vi "Finished Parsing an Array.vi"(11 "JSON Parser in":refnum<class "JSON Parser.lvclass">) -> (3 "JSON Parser out":refnum<class "JSON Parser.lvclass">)   [LabVIEW 2020, in "JKI JSON Serialization.lvlib" / "JSON Parser.lvclass"]
uses:
  JSON Parser.lvclass
  JSON Parser.lvclass/JSON Parser.ctl
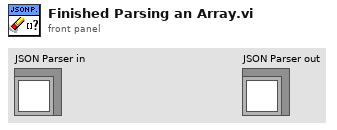
[diagram p1: front panel]
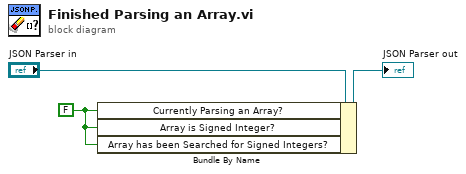
[diagram p0: block diagram]
diagram:
  w1 = FALSE ("Currently Parsing an Array?")
  n1 = Bundle By Name(cluster="JSON Parser in", "Currently Parsing an Array?"=w1, "Array is Signed Integer?"=w1, "Array has been Searched for Signed Integers?"=w1) -> (→"JSON Parser out":refnum<class "JSON Parser.lvclass">)
